vi "2B_Tech Serial Data Recording & DECADE.vi"() -> ()   [LabVIEW 2014]
uses:
  <vilib>/Instr/_visa.llb/VISA Set IO Buffer Mask.ctl
  <vilib>/Instr/_visa.llb/VISA Flush IO Buffer Mask.ctl
  <vilib>/Platform/TimedLoop/XDataNode/timing_clust.ctl
  <vilib>/Platform/TimedLoop/XDataNode/nitl_modes.ctl
  <vilib>/Platform/TimedLoop/XDataNode/wakeup.ctl
  <vilib>/Utility/error.llb/whitespace.ctl
  <vilib>/Instr/_visa.llb/VISA Configure Serial Port (Instr).vi
  <vilib>/Utility/tcp.llb/UDP Multicast Read-Only Open.vi
  <vilib>/Utility/tcp.llb/UDP Multicast Write-Only Open.vi
  <vilib>/platform/TimedLoop/XDataNode/XDataNode.xnode
  <vilib>/Platform/TimedLoop/XDataNode/XDNodeRunTimeDep.lvlib
panel:
  in  "timeout (10sec)":u32=3000
  in  "VISA resource name":refnum<visa-resource-name>="ASRL2::INSTR"
  in  "Ambient or Cabin Mode":bool
  in  "Simulate 3 av":dbl
  in  "Simulate\nConc":i32
  in  "Simulate\nconc":bool
  in  "3hr_alm_thresh":i32=80
  out "3hrAvg_Alarm":bool
  out "Inst_Alarm":bool
  in  "Inst_alm_thresh":i32=220
  out "Time":string
  in  "Clear Display\nErrors":bool
  out "Read Error Counter\nfrom process loop":u32
  out "CABOZO UDP_ASCII_Out":string
  out "Ozo_array":string[](array[string])
  out "3hr_ozo_avg":dbl
  out "q_size":i32
  out "Data Output":string[](array[string])
  out "UDP packet\nSend status":bool
  out "TWBOZO UDP_ASCII_Out":string
  in  "spare_2":string="0"
  in  "spare_1":string="0"
  out "UDP_Out_Error":errorcluster
  out "UDP_Pack_num":u32
  out "UDP_In_Error":errorcluster
  out "UDP_In":string
  in  "stop":bool
  in  "Flight Number":string
  out "Number of times \nRead time out":u32
  out "Data Loop count":i32
  out "2B_Serial_error out":errorcluster
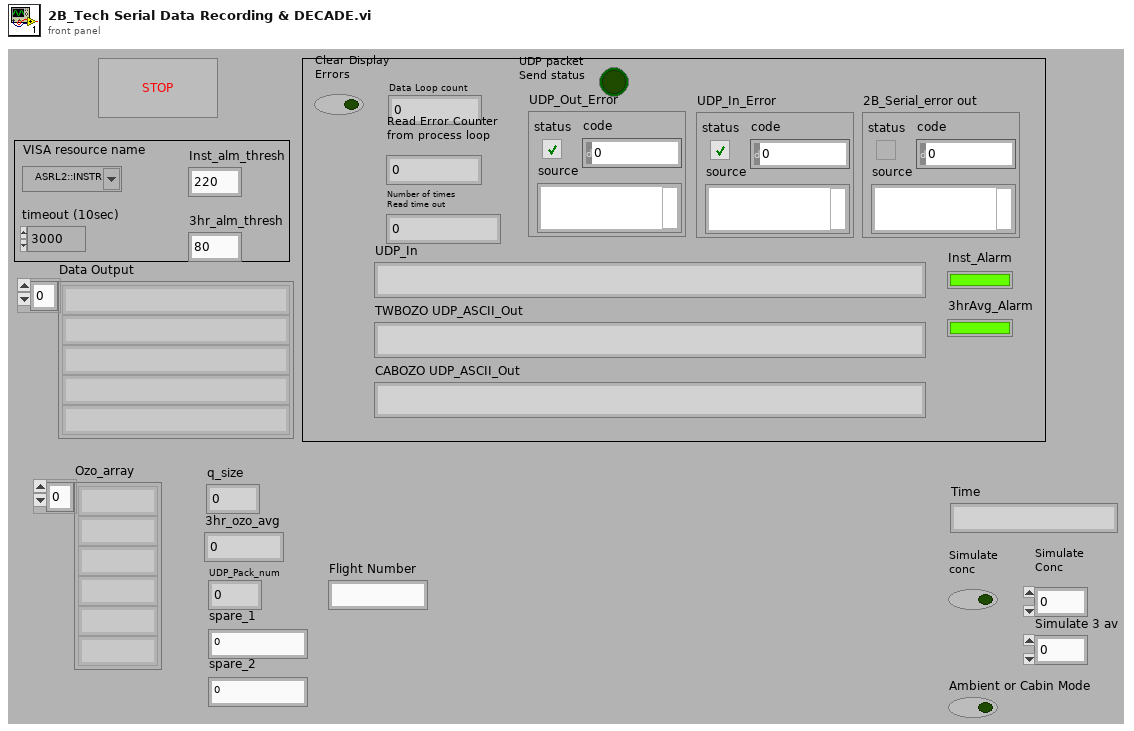
[diagram p1: front panel]
types:
  T1 = typedef "XDNodeRunTimeDep.lvlib/timing_clust.ctl" = cluster{"Expected End [f-1]":u64, "Actual End [f-1]":u64, "Finished Late? [f-1]":bool, "Expected End [i-1]":u64, "Actual End [i-1]":u64, "Finished Late? [i-1]":bool, "Expected Start [i]":u64, "Actual Start [i]":u64, "Expected Start [f]":u64, "Actual Start [f]":u64, "Source Name":string, "Structure Name":string, "Period":i64, "Deadline":i64, "Offset":i64, "Start":i64, "Priority":i32, "Timeout":i32, "Mode":T2, "Wakeup Reason":T3, "Error":errorcluster, "Source Type":string, "Secondary Source Type":string, "Global End Time":u64, "Global Start Time":u64, "Frame Duration":u64, "Iteration Duration":u64, "Assigned CPU":i32, "I/O Scan Engine Mode":u32}
  T2 = typedef "XDNodeRunTimeDep.lvlib/nitl_modes.ctl" = enum32{"No Change", "Process missed periods, maintain original phase", "Discard missed periods, maintain original phase", "Process missed periods, ignore original phase", "Discard missed periods, ignore original phase"}
  T3 = typedef "XDNodeRunTimeDep.lvlib/wakeup.ctl" = enum32{"Normal", "Aborted", "Asynchronous wakeup", "Timing source error", "Timed loop error", "Timeout"}
  T4 = typedef "VISA Flush IO Buffer Mask.ctl" = u16
  T5 = typedef "VISA Set IO Buffer Mask.ctl" = u16
  T6 = typedef "whitespace.ctl" = u16
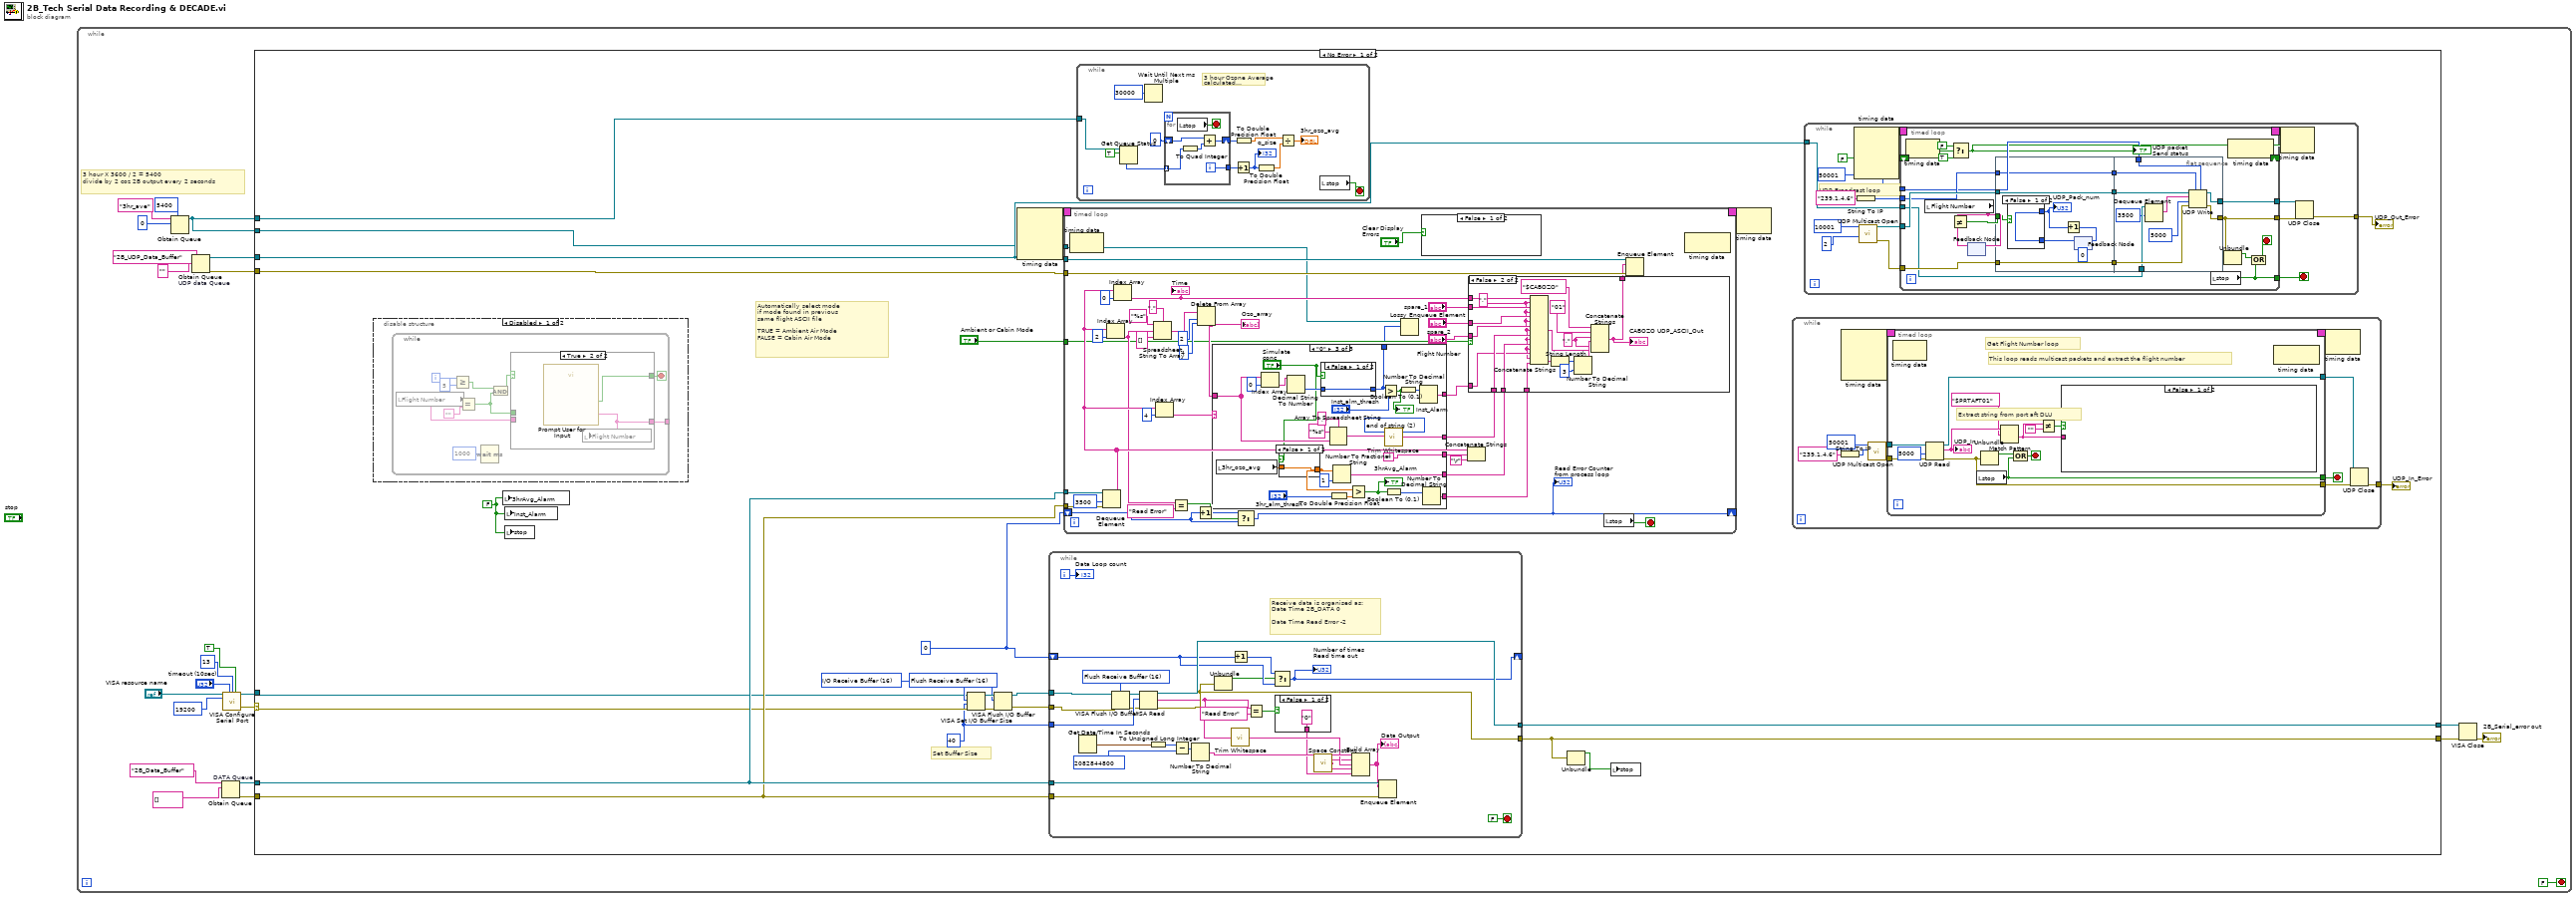
[diagram p0: block diagram]
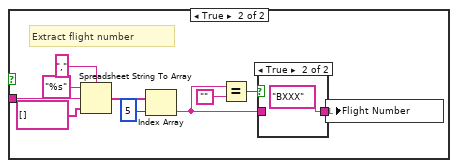
[diagram p2: hidden frame]
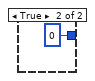
[diagram p4: hidden frame]
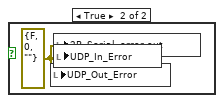
[diagram p5: hidden frame]
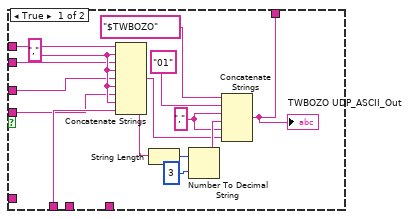
[diagram p6: hidden frame]
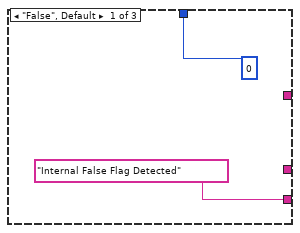
[diagram p7: hidden frame]
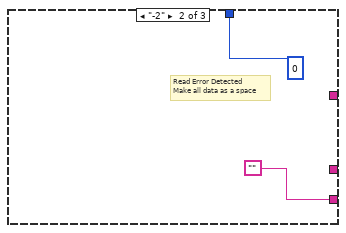
[diagram p8: hidden frame]
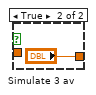
[diagram p9: hidden frame]
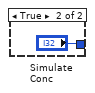
[diagram p10: hidden frame]
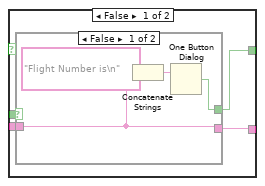
[diagram p11: hidden frame]
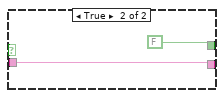
[diagram p12: hidden frame]
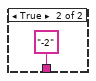
[diagram p14: hidden frame]
diagram:
  n1 = while {
    stop <- FALSE stop-if-true
    # "3 hour X 3600 / 2 = 5400\ndivide by 2 coz 2B output every 2 seconds"
    n2 = Obtain Queue(max queue size (-1, unlimited)=5400, name (unnamed)="3hr_ave", element data type=0 ("index")) -> (queue out=w9:refnum<queue>)  [unwired: 2 in, 2 out]
    n3 = Obtain Queue "UDP data Queue"(name (unnamed)="2B_UDP_Data_Buffer", element data type="") -> (queue out=w15:refnum<queue>, error out=w14:errorcluster)  [unwired: 3 in, 1 out]
    n4 = Obtain Queue "DATA Queue"(name (unnamed)="2B_Data_Buffer", element data type=string[] []) -> (queue out=w19:refnum<queue>, error out=w18:errorcluster)  [unwired: 3 in, 1 out]
    n5 = call-poly "VISA Configure Serial Port"("VISA resource name"="VISA resource name", "timeout (10sec)"="timeout (10sec)", "termination char\n(0xA = '\\n' = LF)"=u8 13 ("termination char\n(0xA = '\\n' = LF)"), "Enable Termination\nChar (T)"=TRUE ("Enable Termination\nChar (T)"), "baud rate (9600)"=u32 19200) -> ("VISA resource name out"=w3:refnum<visa-resource-name>, "error out"=w2:errorcluster)  [unwired: 9 in]
    n6 = case shown="No Error" w2 {
      selector: w2 -> [w34 w326]
      tunnel: w3 -> [w33 w327]
      tunnel: [w48 w327] -> w22
      tunnel: [w31 w326] -> w23
      tunnel: w19 -> [w47 _]
      tunnel: w18 -> [w46 _]
      tunnel: w15 -> [w44 _]
      tunnel: w14 -> [w45 _]
      tunnel: w9 -> [w43 _]
      tunnel: w9 -> [w42 _]
      frame No Error {
        w32 = u32 40 ("size (4096)")
        w37 = T4 16 items=["Flush Receive Buffer"=16, "Write Transmit Buffer to Device"=32, "Flush Receive Buffer (No I/O)"=64, "Flush Transmit Buffer"=128] ("Mask")
        w38 = T5 16 items=["I/O Receive Buffer"=16, "I/O Transmit Buffer"=32, "I/O Receive and Transmit Buffer"=48] ("Mask")
        w29 = FALSE
        w41 = u32 0
        # "Set Buffer Size"
        # "Automatically select mode\nif mode found in previous\nsame flight ASCII file\n\nTRUE = Ambient Air Mode\nFALSE = Cabin Air Mode"
        n7 = disable-structure shown="Disabled" {
          frame Disabled {
            n8 = while {
              tunnel: [w280] -> _
              i -> [w279]
              stop <- w282 stop-if-true
              n9 = local read "Flight Number"() -> (w274:string)
              n10 = Greater Or Equal?(x=w279, y=5) -> (x >= y?=w277:bool)
              n11 = Equal?(x=w274, y="") -> (x = y?=w275:bool)
              n12 = Wait (ms)(milliseconds to wait=u32 1000) -> ()  [unwired: 1 out]
              n13 = And(x=w277, y=w275) -> (x .and. y?=w276:bool)
              n14 = case shown="True" w276 {
                tunnel: [w284 w295] -> w282
                tunnel: [w285 w294] -> w280
                tunnel: w275 -> [w287 _]
                tunnel: w274 -> [w286 _]
                frame False {
                  n15 = case shown="False" w287 {
                    tunnel: [w289 w293] -> w285
                    tunnel: w286 -> [w289 w293]
                    tunnel: [w291 FALSE] -> w284
                    frame False {
                      n16 = Concatenate Strings("Flight Number is\n" ("string"), w289) -> (w288:string)
                      n17 = One Button Dialog(message=w288) -> (true=w291:bool)  [unwired: 1 in]
                    }
                    frame True {
                    }
                  }
                }
                frame True {
                  n18 = call "Prompt User for Input"() -> ("Flight Number BXXX"=w294:string, "OK"=w295:bool)  [unwired: 17 in, 1 out]
                  n19 = local write "Flight Number"(w294) -> ()
                }
              }
            }
          }
          frame Enabled {
          }
        }
        n20 = local write "3hrAvg_Alarm"(w29) -> ()
        n21 = local write "Inst_Alarm"(w29) -> ()
        n22 = local write "stop"(w29) -> ()
        n23 = VISA Set I/O Buffer Size(VISA resource name=w33, mask (16)=w38, size (4096)=w32, error in (no error)=w34) -> (VISA resource name out=w39:refnum<visa-resource-name>, error out=w40:errorcluster)
        n24 = VISA Flush I/O Buffer(VISA resource name=w39, mask (16)=w37, error in (no error)=w40) -> (VISA resource name out=w36:refnum<visa-resource-name>, error out=w35:errorcluster)
        n25 = node-c288() -> (w28:T1)  [unwired: 4 in]
        n26 = while {
          tunnel: [w314] -> w31
          shift-right: [w320] -> _
          shift-left: w41 -> [w321]
          tunnel: [w323] -> w48
          tunnel: w36 -> [w319]
          tunnel: w35 -> [w318]
          tunnel: w47 -> [w317]
          tunnel: w46 -> [w316]
          tunnel: w32 -> [w315]
          i -> [w322]
          stop <- FALSE stop-if-true
          w299 = T4 16 items=["Flush Receive Buffer"=16, "Write Transmit Buffer to Device"=32, "Flush Receive Buffer (No I/O)"=64, "Flush Transmit Buffer"=128] ("Mask")
          # "Receive data is organised as:\nDate Time 2B_DATA 0\n\nDate Time Read Error -2"
          n27 = Get Date/Time In Seconds() -> (seconds since 1Jan1904=w309:timestamp)
          n28 = VISA Flush I/O Buffer(VISA resource name=w319, mask (16)=w299, error in (no error)=w318) -> (VISA resource name out=w300:refnum<visa-resource-name>, error out=w298:errorcluster)
          n29 = VISA Read(VISA resource name=w300, byte count=w315, error in (no error)=w298) -> (VISA resource name out=w323:refnum<visa-resource-name>, read buffer=w297:string, error out=w314:errorcluster)  [unwired: 1 out]
          n30 = To Unsigned Long Integer(number=w309) -> (unsigned 32bit integer=w311:u32)
          n31 = Subtract(x=w311, y=u32 2082844800) -> (x-y=w308:u32)
          n32 = Number To Decimal String(number=w308) -> (decimal integer string=w305:string)  [unwired: 1 in]
          n33 = Unbundle(w314) -> ("status"=w312:bool)  [unwired: 2 out]
          n34 = Increment(x=w321) -> (x+1=w313:u32)
          n35 = call <vilib>:"Trim Whitespace.vi"("string"=w297) -> ("trimmed string"=w304:string)  [unwired: 1 in]
          n36 = Equal?(x=w297, y="Read Error") -> (x = y?=w306:bool)
          n37 = Select(t=w313, s=w312, f=w321) -> (s? t:f=w320:u32)
          "Number of times \nRead time out" <- w320
          n38 = case shown="False" w306 {
            tunnel: ["0" "-2"] -> w302
            frame False {
            }
            frame True {
            }
          }
          n39 = call <vilib>:"Space Constant.vi"() -> ("String"=w303:string)
          n40 = Build Array(w305, w303, w304, w303, w302) -> (w301:string[])
          "Data Output" <- w301
          n41 = Enqueue Element(queue=w317, element=w301, error in (no error)=w316) -> ()  [unwired: 1 in, 3 out]
          "Data Loop count" <- w322
        }
        n42 = timed-loop {
          timing: w28 -> [_]
          timing-out: [_] -> w27
          tunnel: w47 -> [w204]
          tunnel: w46 -> [w203]
          tunnel: w44 -> [w202]
          tunnel: w45 -> [w201]
          tunnel: w42 -> [w167]
          shift-right: [w174] -> _
          shift-left: w41 -> [w175]
          tunnel: "Ambient or Cabin Mode" -> [w173]
          stop <- w169 stop-if-true
          n43 = node-c288() -> ()  [unwired: 1 in, 1 out]
          n44 = Dequeue Element(queue=w204, timeout in ms (-1)=3500, error in (no error)=w203) -> (element=w186:string[])  [unwired: 3 out]
          n45 = Index Array(array=w186, index=2) -> (element=w176:string)
          n46 = Index Array(array=w186, index=0) -> (element=w188:string)
          "Time" <- w188
          n47 = Spreadsheet String To Array(delimiter (Tab)=",", format string="%s", spreadsheet string=w176, array type (2D Dbl)=string[] [] ("Values Array")) -> (array=w193:string[])
          n48 = Index Array(array=w186, index=4) -> (element=w194:string)
          n49 = Equal?(x=w176, y="Read Error") -> (x = y?=w178:bool)
          n50 = Increment(x=w175) -> (x+1=w177:u32)
          n51 = Delete From Array(array=w193, length=2, index=4) -> (array with subset deleted=w190:string[])  [unwired: 1 out]
          "Ozo_array" <- w190
          n52 = case shown="\"0\"" w194 {
            tunnel: w190 -> [_ _ w258]
            tunnel: [_ _ w261] -> w187
            tunnel: [0 0 w244] -> w166
            tunnel: ["Internal False Flag Detected" "" ""] -> w185
            tunnel: [_ _ w255] -> w180
            tunnel: [_ _ w251] -> w171
            tunnel: [_ _ w246] -> w170
            frame "False", Default {
            }
            frame "-2" {
              # "Read Error Detected\nMake all data as a space"
            }
            frame "0" {
              w262 = T6 2 items=["both", "start of string", "end of string"] ("location (both)")
              n53 = local read "3hr_ozo_avg"() -> (w242:dbl)
              n54 = Index Array(array=w258, index=0) -> (element=w259:string)
              n55 = case shown="False" "Simulate\nconc" {
                tunnel: [w266 "Simulate 3 av"] -> w241
                tunnel: w242 -> [w266 _]
                frame False {
                }
                frame True {
                }
              }
              n56 = Decimal String To Number(string=w259) -> (number=w245:i32)  [unwired: 2 in, 1 out]
              n57 = case shown="False" "Simulate\nconc" {
                tunnel: [w268 "Simulate\nConc"] -> w244
                tunnel: w245 -> [w268 _]
                frame False {
                }
                frame True {
                }
              }
              n58 = Array To Spreadsheet String(delimiter (Tab)=",", array=w258, 3:"%s" ("format string")) -> (spreadsheet string=w263:string)
              n59 = To Double Precision Float(number="3hr_alm_thresh") -> (double precision float=w248:dbl)
              n60 = Number To Fractional String(number=w241, precision (6)=i16 1) -> (F-format string=w255:string)  [unwired: 2 in]
              n61 = Greater?(x=w241, y=w248) -> (0:w249:bool)
              "3hrAvg_Alarm" <- w249
              n62 = Greater?(x=w244, y="Inst_alm_thresh") -> (0:w252:bool)
              "Inst_Alarm" <- w252
              n63 = call <vilib>:"Trim Whitespace.vi"("string"=w263, "location (both)"=w262) -> ("trimmed string"=w261:string)
              n64 = Boolean To (0,1)(Boolean=w249) -> (0, 1=w250:i16)
              n65 = Boolean To (0,1)(Boolean=w252) -> (0, 1=w253:i16)
              n66 = Number To Decimal String(number=w253) -> (decimal integer string=w251:string)  [unwired: 1 in]
              n67 = Number To Decimal String(number=w250) -> (decimal integer string=w246:string)  [unwired: 1 in]
            }
          }
          n68 = Select(t=w177, s=w178, f=w175) -> (s? t:f=w174:u32)
          "Read Error Counter\nfrom process loop" <- w174
          n69 = Lossy Enqueue Element(queue=w167, element=w166) -> ()  [unwired: 1 in, 4 out]
          n70 = case shown="False" "Clear Display\nErrors" {
            frame False {
            }
            frame True {
              w205 = errorcluster {"status"=FALSE, "code"=0, "source"=""} ("UDP Error Out")
              n71 = local write "UDP_Out_Error"(w205) -> ()
              n72 = local write "2B_Serial_error out"(w205) -> ()
              n73 = local write "UDP_In_Error"(w205) -> ()
            }
          }
          n74 = Concatenate Strings(w186, w185, "\r") -> ()  [unwired: 1 out]
          n75 = case shown="False" w173 {
            tunnel: [w211 w229] -> w200
            tunnel: w188 -> [w210 w228]
            tunnel: w187 -> [w209 w227]
            tunnel: "spare_1" -> [w208 w226]
            tunnel: "spare_2" -> [w207 w225]
            tunnel: "Flight Number" -> [w206 w224]
            tunnel: w180 -> [_ w223]
            tunnel: w171 -> [_ w222]
            tunnel: w170 -> [_ w220]
            frame True {
              w219 = ","
              w215 = ","
              n76 = Concatenate Strings(w210, w219, w208, w219, w207, w219, w206, w219, w209) -> (w214:string)
              n77 = String Length(string=w214) -> (length=w218:i32)
              n78 = Number To Decimal String(number=w218, width (-)=i16 3) -> (decimal integer string=w216:string)
              n79 = Concatenate Strings("$TWBOZO", "01", w215, w216, w215, w214) -> (w211:string)
              "TWBOZO UDP_ASCII_Out" <- w211
            }
            frame False {
              w221 = ","
              w233 = ","
              n80 = Concatenate Strings(w228, w221, w226, w221, w225, w221, w224, w221, w227, w221, w223, w221, w222, w221, w220) -> (w232:string)
              n81 = String Length(string=w232) -> (length=w236:i32)
              n82 = Number To Decimal String(number=w236, width (-)=i16 3) -> (decimal integer string=w234:string)
              n83 = Concatenate Strings("$CABOZO", "01", w233, w234, w233, w232) -> (w229:string)
              "CABOZO UDP_ASCII_Out" <- w229
            }
          }
          n84 = local read "stop"() -> (w169:bool)
          n85 = Enqueue Element(queue=w202, element=w200, error in (no error)=w201) -> ()  [unwired: 1 in, 3 out]
          n86 = node-c288() -> ()  [unwired: 1 in, 1 out]
        }
        n87 = while {
          tunnel: w43 -> [w52]
          stop <- w54 stop-if-true
          # "3 hour Ozone Average calculated\nevery 30 seconds"
          n88 = Get Queue Status(queue=w52, return elements? (F)=TRUE) -> (elements=w49:i32[])  [unwired: 1 in, 7 out]
          n89 = Wait Until Next ms Multiple(millisecond multiple=u32 30000) -> ()  [unwired: 1 out]
          n90 = for {
            tunnel: [w66] -> w60
            shift-right: [w65] -> w58
            shift-left: i64 0 -> [w64]
            tunnel: w49 -> [w62] mode=indexing
            i -> [w66]
            stop <- w61 stop-if-true
            n91 = local read "stop"() -> (w61:bool)
            n92 = To Quad Integer(1:w62) -> (0:w63:i64)
            n93 = Add(x=w64, y=w63) -> (x+y=w65:i64)
          }
          n94 = Increment(x=w60) -> (x+1=w53:i32)
          "q_size" <- w53
          n95 = To Double Precision Float(number=w58) -> (double precision float=w56:dbl)
          n96 = To Double Precision Float(number=w53) -> (double precision float=w57:dbl)
          n97 = Divide(x=w56, y=w57) -> (x/y=→"3hr_ozo_avg":dbl)
          n98 = local read "stop"() -> (w54:bool)
        }
        n99 = Unbundle(w31) -> ("status"=w30:bool)  [unwired: 2 out]
        n100 = local write "stop"(w30) -> ()
        n101 = node-c288(w27) -> ()  [unwired: 1 out]
        n102 = while {
          tunnel: [w67] -> w24
          stop <- w70 stop-if-true
          n103 = node-c288() -> (w69:T1)  [unwired: 4 in]
          n104 = String To IP(1:"239.1.4.6" ("name")) -> (0:w77:u32)
          n105 = call-poly <vilib>:"UDP Multicast Open.vi"("multicast addr"=w77, "port"=u16 50001) -> ("error out"=w73:errorcluster, "connection ID"=w74:refnum<k16>)  [unwired: 7 in, 1 out]
          n106 = timed-loop {
            tunnel: w74 -> [w90]
            tunnel: w73 -> [w89]
            tunnel: [w84] -> w72
            tunnel: [w82] -> w71
            tunnel: [w80] -> w70
            timing: w69 -> [_]
            timing-out: [_] -> w68
            stop <- w81 stop-if-true
            # "Extract string from port aft DLU"
            # "Get Flight Number loop"
            # "This loop reads multicast packets and extract the flight number"
            n107 = node-c288() -> ()  [unwired: 1 in, 1 out]
            n108 = UDP Read(connection ID=w90, timeout ms (25000)=5000, 8:w89) -> (data out=w85:string, error out=w82:errorcluster, 3:w84:refnum<k16>)  [unwired: 1 in, 2 out]
            "UDP_In" <- w85
            n109 = local read "stop"() -> (w80:bool)
            n110 = Unbundle(w82) -> ("status"=w83:bool)  [unwired: 2 out]
            n111 = Match Pattern(string=w85, regular expression="$PRTAFT01") -> (after substring=w86:string)  [unwired: 1 in, 3 out]
            n112 = Compound Arithmetic op=OR(w83, w80) -> (w81:bool)
            n113 = Not Equal?(x=w86, y="") -> (x != y?=w87:bool)
            n114 = case shown="False" w87 {
              tunnel: w86 -> [_ w97]
              frame False {
              }
              frame True {
                # "Extract flight number"
                n115 = Spreadsheet String To Array(delimiter (Tab)=",", format string="%s", spreadsheet string=w97, array type (2D Dbl)=string[] []) -> (array=w99:string[])
                n116 = Index Array(array=w99, index=5) -> (element=w94:string)
                n117 = Equal?(x=w94, y="") -> (x = y?=w96:bool)
                n118 = case shown="True" w96 {
                  tunnel: [w103 "BXXX"] -> w93
                  tunnel: w94 -> [w103 _]
                  frame False {
                  }
                  frame True {
                  }
                }
                n119 = local write "Flight Number"(w93) -> ()
              }
            }
            n120 = node-c288() -> ()  [unwired: 1 in, 1 out]
          }
          n121 = node-c288(w68) -> ()  [unwired: 1 out]
          n122 = UDP Close(connection ID=w72, 8:w71) -> (error out=w67:errorcluster)  [unwired: 1 out]
        }
        "UDP_In_Error" <- w24
        n123 = while {
          tunnel: w44 -> [w108]
          tunnel: [w107] -> w25
          stop <- w109 stop-if-true
          # "UDP Broadcast loop"
          n124 = node-c288() -> (w111:T1)  [unwired: 4 in]
          n125 = String To IP(1:"239.1.4.6" ("name")) -> (0:w113:u32)
          n126 = call-poly <vilib>:"UDP Multicast Open.vi"("time-to-live (1)"=u16 2, "port"=u16 10001) -> ("error out"=w120:errorcluster, "connection ID"=w121:refnum<k16>)  [unwired: 8 in]
          n127 = timed-loop {
            tunnel: w121 -> [w141]
            tunnel: w120 -> [w140]
            tunnel: [w129] -> w116
            shift-right: [w122] -> _
            shift-left: FALSE -> [w134]
            tunnel: [w127] -> w115
            tunnel: w113 -> [w131]
            tunnel: u16 50001 ("port or service name") -> [w130]
            timing: w111 -> [_]
            timing-out: [_] -> w110
            tunnel: [w123] -> w109
            tunnel: w108 -> [w124]
            stop <- w126 stop-if-true
            n128 = node-c288() -> ()  [unwired: 1 in, 1 out]
            n129 = local read "Flight Number"() -> (w125:string)
            n130 = Select(t=FALSE, s=w134, f=TRUE) -> (s? t:f=w122:bool)
            "UDP packet\nSend status" <- w122
            n131 = feedback-in #1(w125) -> ()
            n132 = feedback #1() -> (w136:string)  [unwired: 1 in]
            n133 = Not Equal?(x=w125, y=w136) -> (x != y?=w135:bool)
            n134 = flat-sequence {
              tunnel: w131 -> [w149]
              tunnel: w140 -> [w150]
              tunnel: w141 -> [w151]
              tunnel: [w151] -> w139
              tunnel: [w150] -> w138
              tunnel: [w149] -> w137
              tunnel: w135 -> [w148]
              tunnel: w130 -> [w163]
              tunnel: w139 -> [w162]
              tunnel: w138 -> [w161]
              tunnel: w137 -> [w160]
              tunnel: [w159] -> w129
              tunnel: [w158] -> w127
              tunnel: w124 -> [w156]
              frame #0 {
                n135 = feedback #2(u32 0) -> (w145:u32)
                n136 = case shown="False" w148 {
                  tunnel: w145 -> [w152 _]
                  tunnel: [w152 u32 0] -> w144
                  frame False {
                  }
                  frame True {
                  }
                }
                "UDP_Pack_num" <- w144
                n137 = Increment(x=w144) -> (x+1=w146:u32)
                n138 = feedback-in #2(w146) -> ()
              }
              frame #1 {
                n139 = Dequeue Element(queue=w156, timeout in ms (-1)=3500) -> (element=w157:string)  [unwired: 1 in, 3 out]
                n140 = UDP Write(address=w160, port or service name=w163, connection ID=w162, data in=w157, 8:w161, 9:5000 ("timeout ms (25000)")) -> (error out=w158:errorcluster, 3:w159:refnum<k16>)
              }
            }
            n141 = local read "stop"() -> (w123:bool)
            n142 = Unbundle(w127) -> ("status"=w128:bool)  [unwired: 2 out]
            n143 = node-c288() -> ()  [unwired: 1 in, 1 out]
            n144 = Compound Arithmetic op=OR(w128, w123) -> (w126:bool)
          }
          n145 = node-c288(w110) -> ()  [unwired: 1 out]
          n146 = UDP Close(connection ID=w116, 8:w115) -> (error out=w107:errorcluster)  [unwired: 1 out]
        }
        "UDP_Out_Error" <- w25
      }
      frame Error {
      }
    }
    n147 = VISA Close(VISA resource name=w22, error in (no error)=w23) -> (error out=→"2B_Serial_error out":errorcluster)
  }
